vi "Test Time to string.vi"(8 "error in (no error)":errorcluster, 11 "TestCase in":refnum<class "Unit Testing.lvclass">) -> (0 "error out":errorcluster, 3 "TestCase out":refnum<class "Unit Testing.lvclass">)   [LabVIEW 2020, in "Unit Testing.lvclass"]
uses:
  Unit Testing.lvclass
  <vilib>/addons/_JKI Toolkits/VI Tester/TestCase.llb/TestCase.lvclass
  Contabilidad/Contabilidad.lvlib
  C:/Program Files (x86)/National Instruments/LabVIEW 2020/vi.lib/addons/_JKI Toolkits/VI Tester/TestCase.llb/TestCase.lvclass
panel:
  in  "Time":timestamp
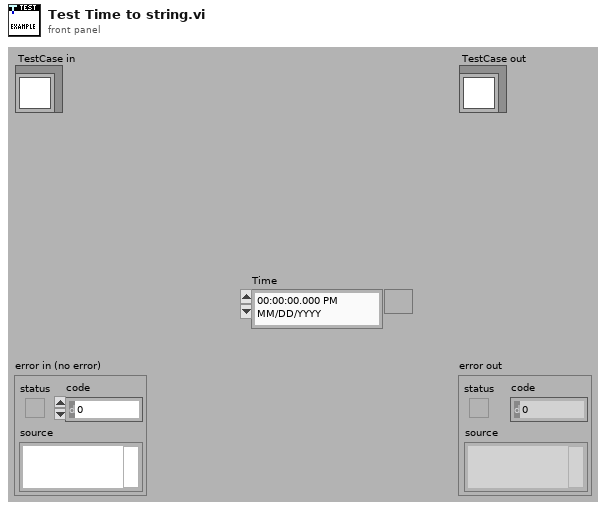
[diagram p1: front panel]
types:
  T1 = typedef "LVDateTimeRec.ctl" = cluster{"fractional second":dbl, "second":i32, "minute":i32, "hour":i32, "day of month":i32, "month":i32, "year":i32, "day of week":i32, "day of year":i32, "DST":i32}
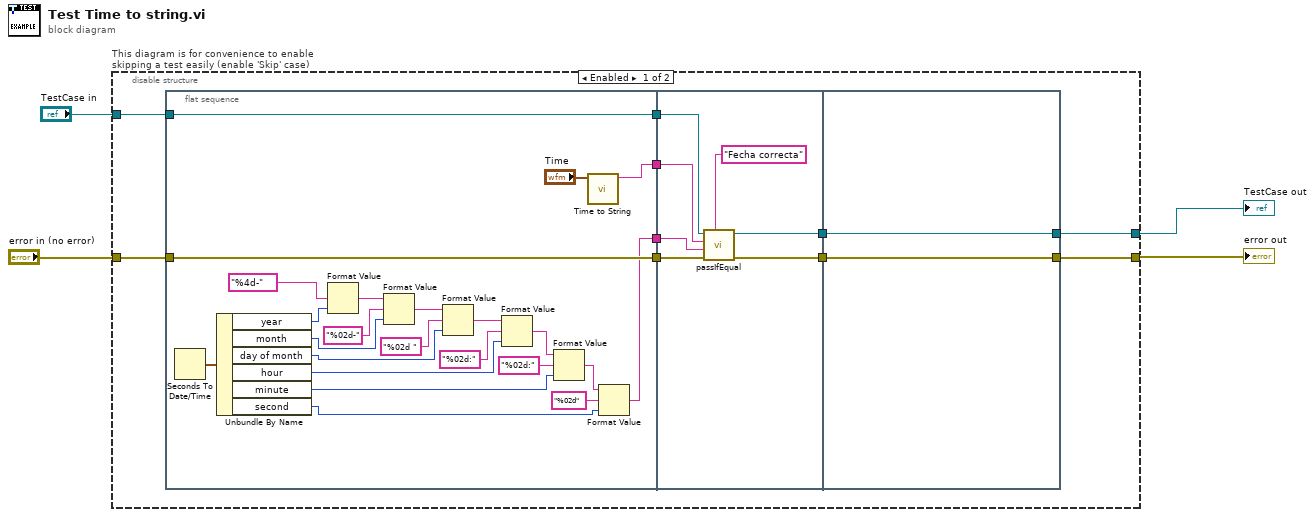
[diagram p0: block diagram]
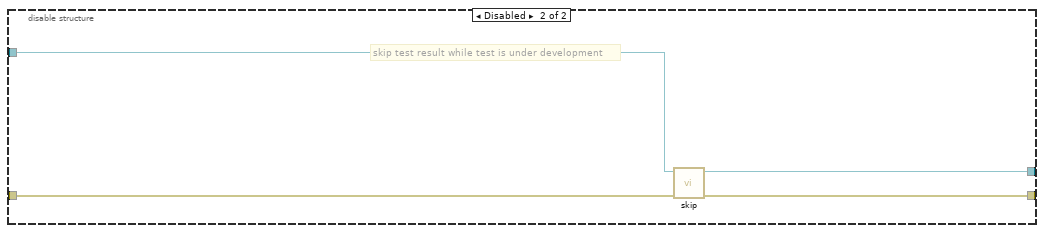
[diagram p2: hidden frame]
diagram:
  n1 = disable-structure "This diagram is for convenience to enable skipping a test easily (enable 'Skip' case)" shown="Enabled" {
    disable-tunnel: "TestCase in" -> [w8 w50]
    disable-tunnel: [w5 w48] -> w1
    disable-tunnel: [w6 w49] -> w3
    disable-tunnel: "error in (no error)" -> [w7 w47]
    frame Enabled {
      n2 = flat-sequence {
        tunnel: [w37] -> w14
        tunnel: w8 -> [w37]
        tunnel: [w36] -> w13
        tunnel: w7 -> [w36]
        tunnel: [w35] -> w12
        tunnel: [w15] -> w11
        tunnel: w14 -> [w44]
        tunnel: w13 -> [w43]
        tunnel: [w42] -> w10
        tunnel: [w41] -> w9
        tunnel: w12 -> [w40]
        tunnel: w11 -> [w39]
        tunnel: w10 -> [w46]
        tunnel: [w46] -> w6
        tunnel: [w45] -> w5
        tunnel: w9 -> [w45]
        frame #0 {
          n3 = Seconds To Date/Time() -> (date time rec=w16:T1)  [unwired: 2 in]
          n4 = Unbundle By Name(w16) -> ("year"=w29:i32, "month"=w30:i32, "day of month"=w31:i32, "hour"=w17:i32, "minute"=w20:i32, "second"=w21:i32)
          n5 = Format Value(format string="%4d-", value (0)=w29) -> (output string=w26:string)  [unwired: 1 in]
          n6 = Format Value(string ("")=w26, format string="%02d-", value (0)=w30) -> (output string=w27:string)
          n7 = Format Value(string ("")=w27, format string="%02d ", value (0)=w31) -> (output string=w28:string)
          n8 = Format Value(string ("")=w28, format string="%02d:", value (0)=w17) -> (output string=w18:string)
          n9 = Format Value(string ("")=w18, format string="%02d:", value (0)=w20) -> (output string=w19:string)
          n10 = call "Time to String.vi"("Time"="Time") -> ("date/time string"=w35:string)  [unwired: 10 in]
          n11 = Format Value(string ("")=w19, format string="%02d", value (0)=w21) -> (output string=w15:string)
        }
        frame #1 {
          n12 = call-dynamic "passIfEqual.vi"("custom report message (\"\")"="Fecha correcta" ("custom report message (\"\")"), "error in (no error)"=w43, "y"=w39, "x"=w40, "TestCase in"=w44) -> ("error out"=w42:errorcluster, "TestCase out"=w41:refnum<class "Unit Testing.lvclass">)  [unwired: 5 in]
        }
        frame #2 {
        }
      }
    }
    frame Disabled {
      # "skip test result while test is under development"
      n13 = call <vilib>:"skip.vi"("error in (no error)"=w47, "TestCase in"=w50) -> ("error out"=w49:errorcluster, "TestCase out"=w48:refnum<class "Unit Testing.lvclass">)  [unwired: 8 in]
    }
  }
  "error out" <- w3
  "TestCase out" <- w1
